vi "Read nodes.vi"(9 "VI_AST in":refnum<class "VI_AST.lvclass">) -> (3 "VI_AST out":refnum<class "VI_AST.lvclass">, 4 "nodes":i32[](array[numeric]))   [LabVIEW 2014, in "VI_AST.lvclass"]
uses:
  VI_AST.lvclass
  VI_AST.lvclass/VI_AST.ctl
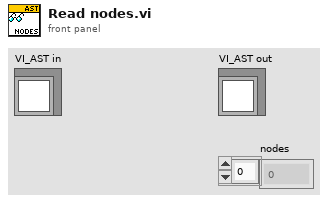
[diagram p1: front panel]
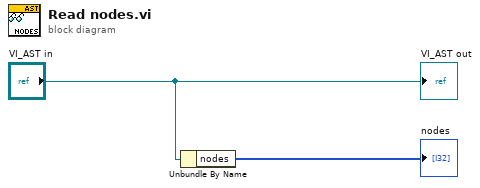
[diagram p0: block diagram]
diagram:
  n1 = Unbundle By Name("VI_AST in") -> ("nodes"=→"nodes":i32[])
  "VI_AST out" <- "VI_AST in"
